vi "State Exit.vi"(11 "Msging Self Actor State in":refnum<class "Msging Self Actor State.lvclass">) -> (0 "error out":errorcluster, 3 "Msging Self Actor State out":refnum<class "Msging Self Actor State.lvclass">)   [LabVIEW 2021, in "LVCAM.lvlib" / "Msging Self Actor State.lvclass"]
uses:
  Msging Self Actor State.lvclass
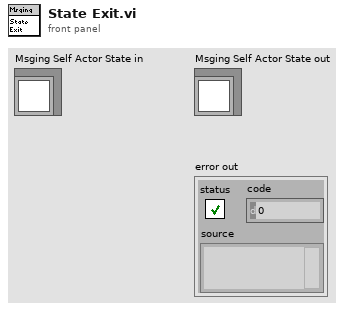
[diagram p1: front panel]
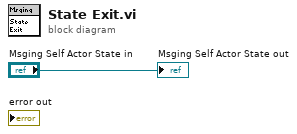
[diagram p0: block diagram]
diagram:
  "Msging Self Actor State out" <- "Msging Self Actor State in"
